vi "Read.vi"(8 "error in (no error)":errorcluster, 9 "Bytes To Read":u8, 10 "Registers":u8[](array[numeric])=[0], 11 "BME68x in":refnum<class "BME680.lvclass">) -> (0 "error out":errorcluster, 2 "Data out":u8[](array[numeric]), 3 "BME68x out":refnum<class "BME680.lvclass">)   [LabVIEW 2022 SP3, in "BME680.lvlib" / "BME680.lvclass"]
uses:
  BME680.lvclass
  BME680.lvclass/BME680.ctl
  <vilib>/MakerHub/LINX/LMH-LINX.lvlib
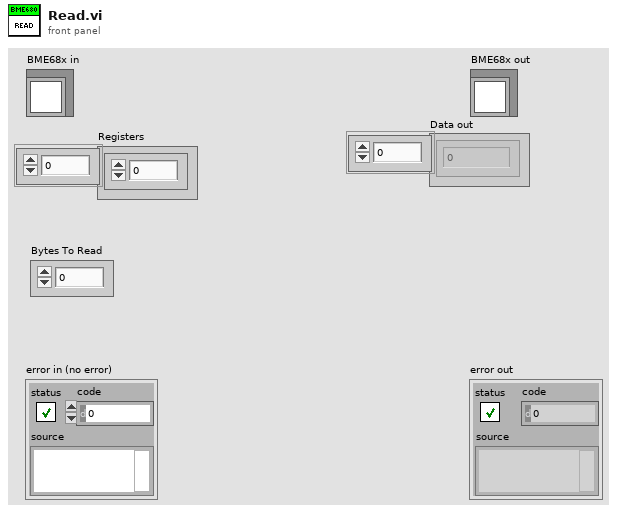
[diagram p1: front panel]
types:
  T1 = typedef "LMH-LINX.lvlib/LINX Ref.ctl" = cluster{"IO":T2, "Interface":T3, "LINX Device Config":T4}
  T2 = typedef "LMH-LINX.lvlib/Platform.ctl" = enum16{"Remote", "Local"}
  T3 = typedef "LMH-LINX.lvlib/Interface.ctl" = enum16{"Serial", "TCP"}
  T4 = typedef "LMH-LINX.lvlib/Device.lvlib/LINX Device Config.ctl" = cluster{"Interface":T3, "COM Port":refnum<visa-resource-name>, "TCP Configuration":T5, "Device Family":u8, "Device ID":u8, "Device Name":string, "TCP Ref":refnum<k5>, "Channels":T6}
  T5 = typedef "LMH-LINX.lvlib/Device.lvlib/TCP Config.ctl" = cluster{"IP Address":string, "Port":u16}
  T6 = typedef "LMH-LINX.lvlib/Channels.ctl" = cluster{"DI":u8[], "DO":u8[], "AI":u8[], "AO":u8[], "PWM":u8[], "QE":u8[], "UART":u8[], "I2C 2":u8[], "SPI":u8[], "CAN":u8[], "Servo":u8[], "AI Ref (V)":dbl, "AI Resolution (Bits)":u8, "AO Ref (V)":dbl, "AO Resolution (Bits)":u8}
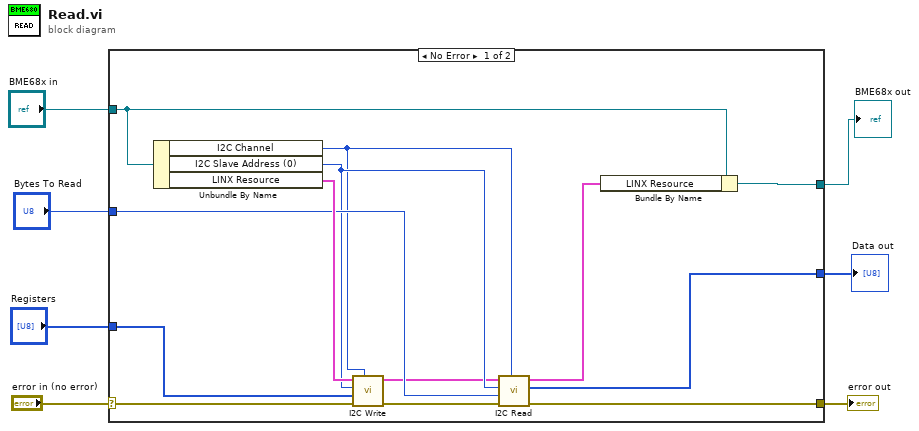
[diagram p0: block diagram]
diagram:
  n1 = case shown="No Error" "error in (no error)" {
    selector: "error in (no error)" -> [w18 w21]
    tunnel: "Registers" -> [w17 _]
    tunnel: "Bytes To Read" -> [w13 _]
    tunnel: "BME68x in" -> [w19 w22]
    tunnel: [w20 w22] -> w3
    tunnel: [w8 _] -> w2
    tunnel: [w15 w21] -> w1
    frame No Error {
      n2 = Unbundle By Name(w19) -> ("I2C Channel"=w10:u8, "I2C Slave Address (0)"=w12:u8, "LINX Resource"=w16:T1)
      n3 = call <vilib>:"I2C Write.vi"("I2C Channel"=w10, "Error In"=w18, "Data"=w17, "I2C Slave Address (0)"=w12, "LINX Resource"=w16) -> ("Error Out"=w14:errorcluster, "LINX Resource"=w11:T1)  [unwired: 5 in]
      n4 = call <vilib>:"I2C Read.vi"("I2C Channel"=w10, "Error In"=w14, "Bytes To Read"=w13, "I2C Slave Address (0)"=w12, "LINX Resource"=w11) -> ("Error Out"=w15:errorcluster, "Data"=w8:u8[], "LINX Resource"=w9:T1)  [unwired: 4 in]
      n5 = Bundle By Name(cluster=w19, "LINX Resource"=w9) -> (w20:refnum<class "BME680.lvclass">)
    }
    frame Error {
    }
  }
  "error out" <- w1
  "BME68x out" <- w3
  "Data out" <- w2
